vi "Load Device Image.vi"(8 "Error In":errorcluster, 10 "Device Index":i32, 11 "Device Family Index":i32) -> (0 "Error Out":errorcluster, 1 "Image Found?":bool, 3 "Device Image":picture)   [LabVIEW 2011, in "LMH-LINX.lvlib"]
doc: "Load LINX Device Image"
uses:
  LMH-LINX.lvlib
  Type Defs/All Firmware Data FGV States.ctl
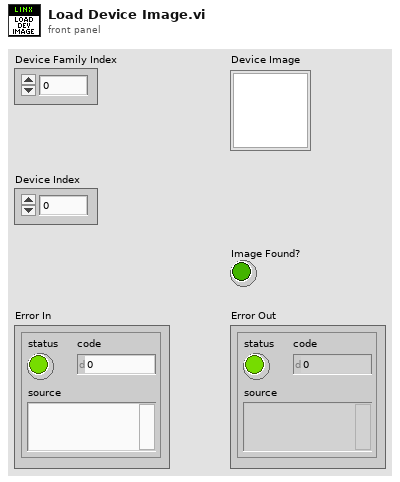
[diagram p1: front panel]
types:
  T1 = typedef "LMH-LINX.lvlib/All Firmware Data FGV States.ctl" = enum16{"Set", "Get"}
  T2 = typedef "LMH-LINX.lvlib/Device Data.ctl" = cluster{"Family ID":i32, "Family Name":string, "Device ID":i32, "Device Name":string, "Firmware Program Interfaces":string[], "Path":path}
  T3 = typedef "imagedata.ctl" = cluster{"image type":i32, "image depth":i32, "image":u8[], "mask":u8[], "colors":u32[], "Rectangle":cluster{"left":i16, "top":i16, "right":i16, "bottom":i16}}
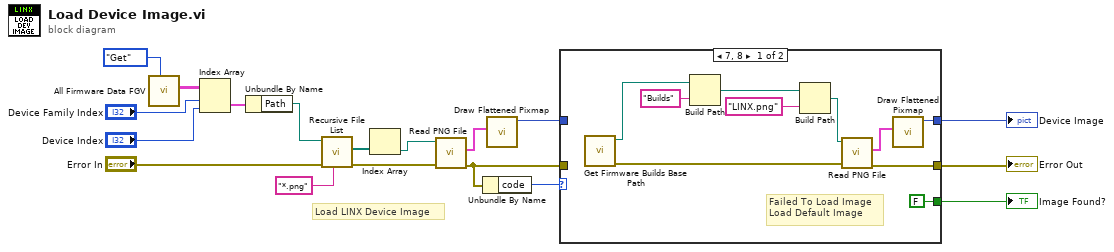
[diagram p0: block diagram]
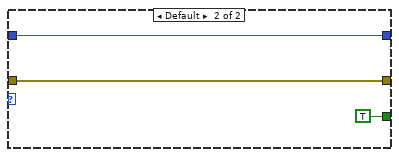
[diagram p2: hidden frame]
diagram:
  # "Load LINX Device Image"
  n1 = call "All Firmware Data FGV.vi"("All Firmware Data FGV States"=All_Firmware_Data_FGV_States."Get") -> ("Devices"=w13:T2[][])  [unwired: 7 in, 3 out]
  n2 = Index Array(array=w13, index (row)="Device Family Index", index (col)="Device Index") -> (element=w9:T2)
  n3 = Unbundle By Name(w9) -> ("Path"=w8:path)
  n4 = call <vilib>:"Recursive File List.vi"("pattern"="*.png", "error in (no error)"="Error In", "Folder Path"=w8) -> ("error out"=w4:errorcluster, "All Files in Dir"=w6:path[])  [unwired: 4 in, 3 out]
  n5 = Index Array(array=w6) -> (element=w5:path)  [unwired: 1 in]
  n6 = call <vilib>:"Read PNG File.vi"("error in (no error)"=w4, "path to PNG file"=w5) -> ("error out"=w1:errorcluster, "image data"=w18:T3)  [unwired: 7 in, 1 out]
  n7 = Unbundle By Name(w1) -> ("code"=w2:i32)
  n8 = call <vilib>:"Draw Flattened Pixmap.vi"("image data"=w18) -> ("new picture"=w16:picture)  [unwired: 8 in]
  n9 = case shown="7, 8" w2 {
    tunnel: [w25 w29] -> w3
    tunnel: [w26 w31] -> w17
    tunnel: w16 -> [_ w31]
    tunnel: [FALSE TRUE] -> w15
    tunnel: w1 -> [_ w29]
    frame 7, 8 {
      # "Failed To Load Image\nLoad Default Image"
      n10 = call "Get Firmware Builds Base Path.vi"() -> ("Error Out"=w22:errorcluster, "Firmware Builds Base Path"=w21:path)  [unwired: 10 in]
      n11 = Build Path(base path=w21, name or relative path="Builds") -> (appended path=w20:path)
      n12 = Build Path(base path=w20, name or relative path="LINX.png") -> (appended path=w24:path)
      n13 = call <vilib>:"Read PNG File.vi"("error in (no error)"=w22, "path to PNG file"=w24) -> ("error out"=w25:errorcluster, "image data"=w28:T3)  [unwired: 7 in, 1 out]
      n14 = call <vilib>:"Draw Flattened Pixmap.vi"("image data"=w28) -> ("new picture"=w26:picture)  [unwired: 8 in]
    }
    frame Default {
    }
  }
  "Error Out" <- w3
  "Device Image" <- w17
  "Image Found?" <- w15
